vi "PRL Check for bad dt.vi"(11 "Timestamp":timestamp[](array[timestamp])) -> (3 "Bad dt":bool)   [LabVIEW 2012, in "PMU Recorder Light.lvlib"]
uses:
  PMU Recorder Light.lvlib
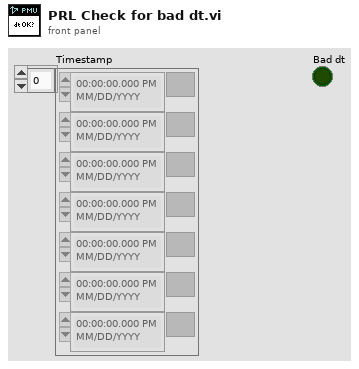
[diagram p1: front panel]
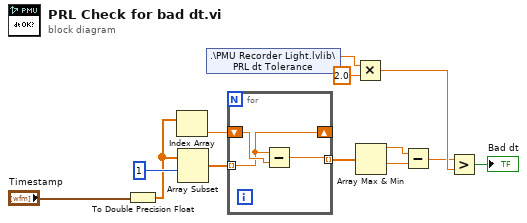
[diagram p0: block diagram]
diagram:
  n1 = To Double Precision Float(number="Timestamp") -> (double precision float=w3:dbl[])
  n2 = Index Array(array=w3) -> (element=w2:dbl)  [unwired: 1 in]
  n3 = Array Subset(array=w3, index=1) -> (w5:dbl[])  [unwired: 1 in]
  n4 = shared-variable ".\\PMU Recorder Light.lvlib\\PRL dt Tolerance"() -> (w8:dbl)  [unwired: 1 in, 1 out]
  n5 = for {
    shift-right: [w14] -> _
    shift-left: w2 -> [w16]
    tunnel: w5 -> [w14] mode=indexing
    tunnel: [w15] -> w6 mode=indexing
    n6 = Subtract(x=w14, y=w16) -> (x-y=w15:dbl)
  }
  n7 = Multiply(x=w8, y=2.0) -> (x*y=w12:dbl)
  n8 = Array Max & Min(array=w6) -> (max value=w7:dbl, min value=w10:dbl)  [unwired: 2 out]
  n9 = Subtract(x=w7, y=w10) -> (x-y=w11:dbl)
  n10 = Greater?(x=w11, y=w12) -> (0:→"Bad dt":bool)
